vi "ProcessData.vi"() -> ()   [LabVIEW 2019]
panel:
  out "Digital":dbl
  out "Drehmoment":dbl
  out "Status/Fehler":dbl
  out "Istgeschwindigkeit":dbl
  out "Handshake":bool
  out "Standby aktiv":bool
  out "Reserviert":bool
  out "SWES inaktiv":bool
  out "Geschwindigkeit erreicht":bool
  out "AS2 aktiv":bool
  out "Warnung":bool
  out "Fehler":bool
  out "in Position":bool
  out "Relativposition übernommen":bool
  out "referenziert":bool
  out "Motor dreht":bool
  out "Bremse geönnet":bool
  out "Endstufenfreigabe":bool
  out "STO inaktiv":bool
  out "Betriebsbereit":bool
  in  "Stopp":bool
  in  "Update(ms)":dbl
  in  "Timeout (ms)":dbl
  in  "IP-Adresse":string
  in  "Digital":dbl
  in  "Deceleration":dbl
  in  "Acceleration":dbl
  in  "Speed":dbl
  in  "Handshake":bool
  in  "Standby":bool
  in  "Inhibit":bool
  in  "Reserviert":bool
  in  "Reservier":bool
  in  "AS2 aktivieren":bool
  in  "Reserviert":bool
  in  "Fehler_Reset":bool
  in  "Start":bool
  in  "Reserviert":bool
  in  "Reserviert":bool
  in  "Reserviert":bool
  in  "Bremse öffnen":bool
  in  "Reserviert":bool
  in  "Enable/ApplicationStop":bool
  in  "Enable/EmergencyStop":bool
  # "zum MOVIDRIVE"
  # "vom MOVIDRIVE"
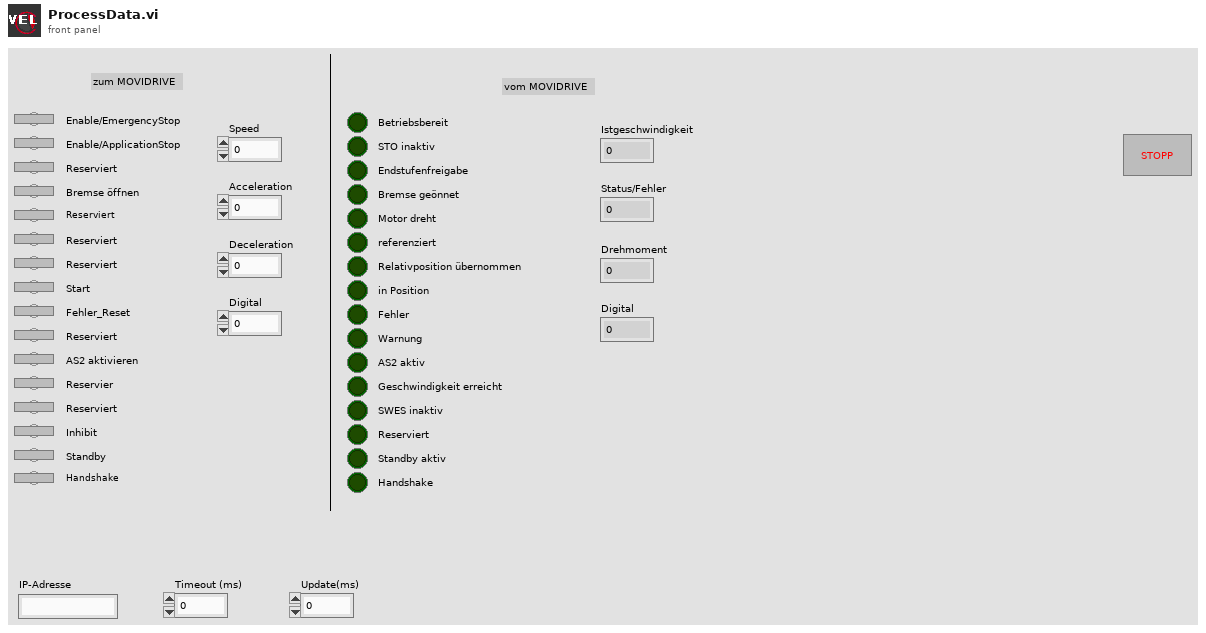
[diagram p1: front panel]
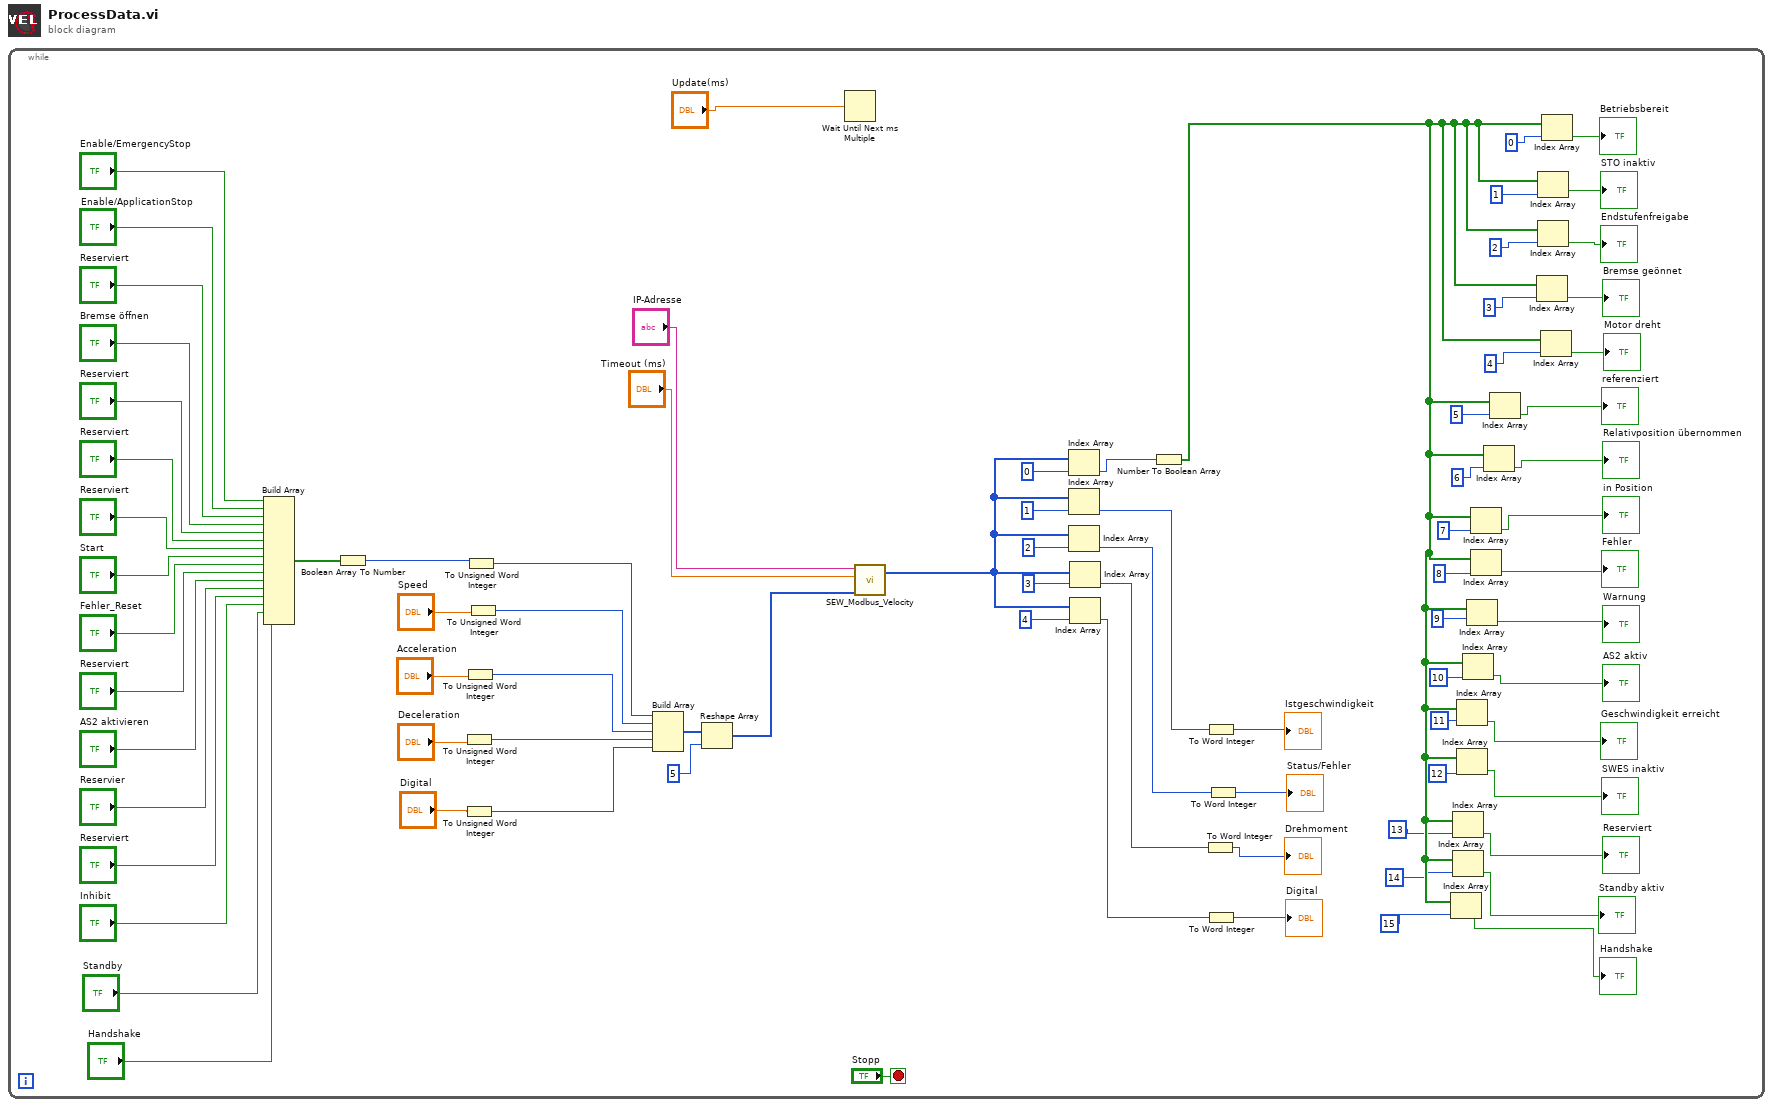
[diagram p0: block diagram]
diagram:
  n1 = while {
    stop <- "Stopp" stop-if-true
    n2 = Build Array("Enable/EmergencyStop", "Enable/ApplicationStop", "Reserviert", "Bremse öffnen", "Reserviert", "Reserviert", "Reserviert", "Start", "Fehler_Reset", "Reserviert", "AS2 aktivieren", "Reservier", "Reserviert", "Inhibit", "Standby", "Handshake") -> (w70:bool[])
    n3 = Boolean Array To Number(Boolean array=w70) -> (number=w71:u32)
    n4 = To Unsigned Word Integer(number="Deceleration") -> (unsigned 16bit integer=w77:u16)
    n5 = To Unsigned Word Integer(number="Digital") -> (unsigned 16bit integer=w78:u16)
    n6 = To Unsigned Word Integer(number="Acceleration") -> (unsigned 16bit integer=w76:u16)
    n7 = To Unsigned Word Integer(number=w71) -> (unsigned 16bit integer=w75:u16)
    n8 = To Unsigned Word Integer(number="Speed") -> (unsigned 16bit integer=w80:u16)
    n9 = Build Array(w75, w80, w76, w77, w78) -> (w81:u16[])
    n10 = Reshape Array(w81, 5) -> (w50:u16[])
    n11 = Wait Until Next ms Multiple(millisecond multiple="Update(ms)") -> ()  [unwired: 1 out]
    n12 = call "SEW_Modbus_Velocity.vi"("Remote IP Address"="IP-Adresse", "Timeout [ms]"="Timeout (ms)", "Output (Write Multiple Register) 2"=w50) -> ("Input (Read Holding Register) 2"=w48:u16[])  [unwired: 3 in]
    n13 = Index Array(array=w48, index=0) -> (element=w34:u16)
    n14 = Index Array(array=w48, index=1) -> (element=w35:u16)
    n15 = Index Array(array=w48, index=2) -> (element=w36:u16)
    n16 = Index Array(array=w48, index=3) -> (element=w37:u16)
    n17 = Index Array(array=w48, index=4) -> (element=w38:u16)
    n18 = Number To Boolean Array(number=w34) -> (Boolean array=w17:bool[])
    n19 = To Word Integer(number=w37) -> (16bit integer=→"Drehmoment":i16)
    n20 = To Word Integer(number=w35) -> (16bit integer=→"Istgeschwindigkeit":i16)
    n21 = To Word Integer(number=w38) -> (16bit integer=→"Digital":i16)
    n22 = To Word Integer(number=w36) -> (16bit integer=→"Status/Fehler":i16)
    n23 = Index Array(array=w17, index=15) -> (element=→"Handshake":bool)
    n24 = Index Array(array=w17, index=13) -> (element=→"Reserviert":bool)
    n25 = Index Array(array=w17, index=14) -> (element=→"Standby aktiv":bool)
    n26 = Index Array(array=w17, index=11) -> (element=→"Geschwindigkeit erreicht":bool)
    n27 = Index Array(array=w17, index=12) -> (element=→"SWES inaktiv":bool)
    n28 = Index Array(array=w17, index=10) -> (element=→"AS2 aktiv":bool)
    n29 = Index Array(array=w17, index=9) -> (element=→"Warnung":bool)
    n30 = Index Array(array=w17, index=7) -> (element=→"in Position":bool)
    n31 = Index Array(array=w17, index=8) -> (element=→"Fehler":bool)
    n32 = Index Array(array=w17, index=6) -> (element=→"Relativposition übernommen":bool)
    n33 = Index Array(array=w17, index=5) -> (element=→"referenziert":bool)
    n34 = Index Array(array=w17, index=3) -> (element=→"Bremse geönnet":bool)
    n35 = Index Array(array=w17, index=1) -> (element=→"STO inaktiv":bool)
    n36 = Index Array(array=w17, index=2) -> (element=→"Endstufenfreigabe":bool)
    n37 = Index Array(array=w17, index=4) -> (element=→"Motor dreht":bool)
    n38 = Index Array(array=w17, index=0) -> (element=→"Betriebsbereit":bool)
  }
